vi "LoadFromConfig.vi"(0 "Array":refnum<vi>[](array[refnum]), 1 "Section":string, 2 "VI Path":path) -> ()   [LabVIEW 2016]
uses:
  <vilib>/Utility/config.llb/Read Key (Double).vi
  <vilib>/Utility/config.llb/NI_LVConfig.lvlib
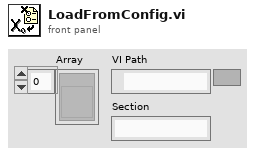
[diagram p1: front panel]
types:
  T1 = typedef "NI_LVConfig.lvlib/Config Data RefNum.ctl" = refnum<k1>
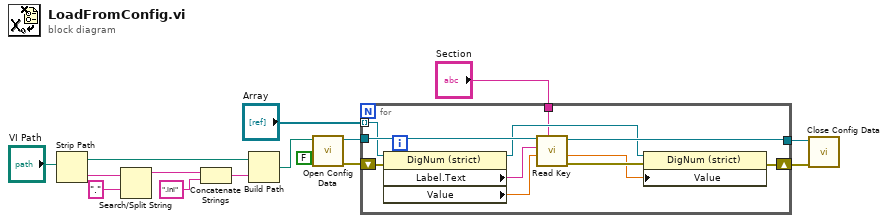
[diagram p0: block diagram]
diagram:
  n1 = Strip Path(path="VI Path") -> (stripped path=w5:path, name=w10:string)
  n2 = Search/Split String(string=w10, search string/char (-)=".") -> (substring before match=w7:string)  [unwired: 1 in, 2 out]
  n3 = Concatenate Strings(w7, ".ini" ("string")) -> (w8:string)
  n4 = Build Path(base path=w5, name or relative path=w8) -> (appended path=w4:path)
  n5 = call <vilib>:"Open Config Data.vi"("create file if necessary (T)"=FALSE, "configuration file path"=w4) -> ("error out"=w14:errorcluster, "refnum"=w15:T1)  [unwired: 7 in, 1 out]
  n6 = for {
    tunnel: w15 -> [w20]
    shift-right: [w25] -> w12
    shift-left: w14 -> [w26]
    tunnel: [w23] -> w13
    tunnel: "Array" -> [w17] mode=indexing
    tunnel: "Section" -> [w16]
    n7 = property class="DigNum (strict)"(reference=w17, error in=w26) -> (reference out=w18:refnum<vi>, "Label.Text"=w19:string, "Value"=w21:dbl)  [unwired: 1 out]
    n8 = call-poly <vilib>:"Read Key.vi"("section"=w16, "default value"=w21, "key"=w19, "refnum"=w20) -> ("error out"=w24:errorcluster, "value"=w22:dbl, "refnum out"=w23:T1)  [unwired: 4 in, 1 out]
    n9 = property class="DigNum (strict)"(reference=w18, error in=w24, "Value"=w22) -> (error out=w25:errorcluster)  [unwired: 1 out]
  }
  n10 = call <vilib>:"Close Config Data.vi"("error in (no error)"=w12, "refnum"=w13) -> ()  [unwired: 8 in, 2 out]
